vi "Elavator_Motor_Value.vi"(6 "Ele_Pos":dbl, 8 "Pos_Des":dbl, 9 "Pos_Active":bool, 11 "Ele_Manual":dbl) -> (2 "Ele_At_Pos":bool, 3 "Ele_Lift_Power":dbl)   [LabVIEW 2014]
panel:
  in  "lower limit":dbl=8.25
  in  "upper limit":dbl=53.5
  out "Pos_Power_Map":cluster{"Speed X":dbl[], "Speed Y":dbl[]}(graph)
  in  "Y_Array":dbl[](array[numeric])=[1.0, 0.15, 0.15, 0.0, -0.15, -0.15, -1.0] format="%.2f"
  in  "X_Array":dbl[](array[numeric])=[-1.75, -0.1, -0.01, 0.0, 0.01, 0.1, 1.75, 0.0, 0.0, 0.0, 100.0] format="%.2f"
  out "y_out":dbl
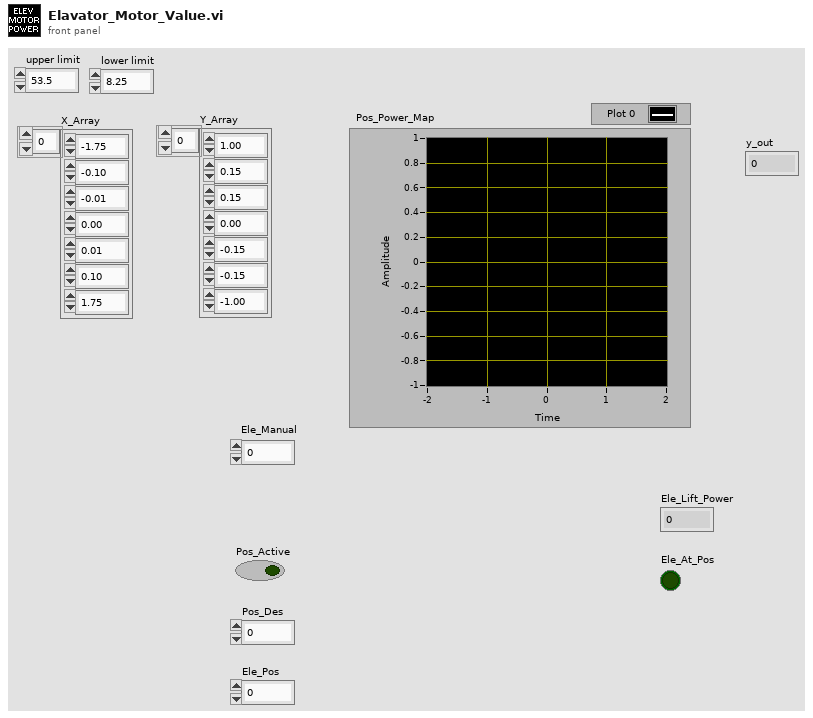
[diagram p1: front panel]
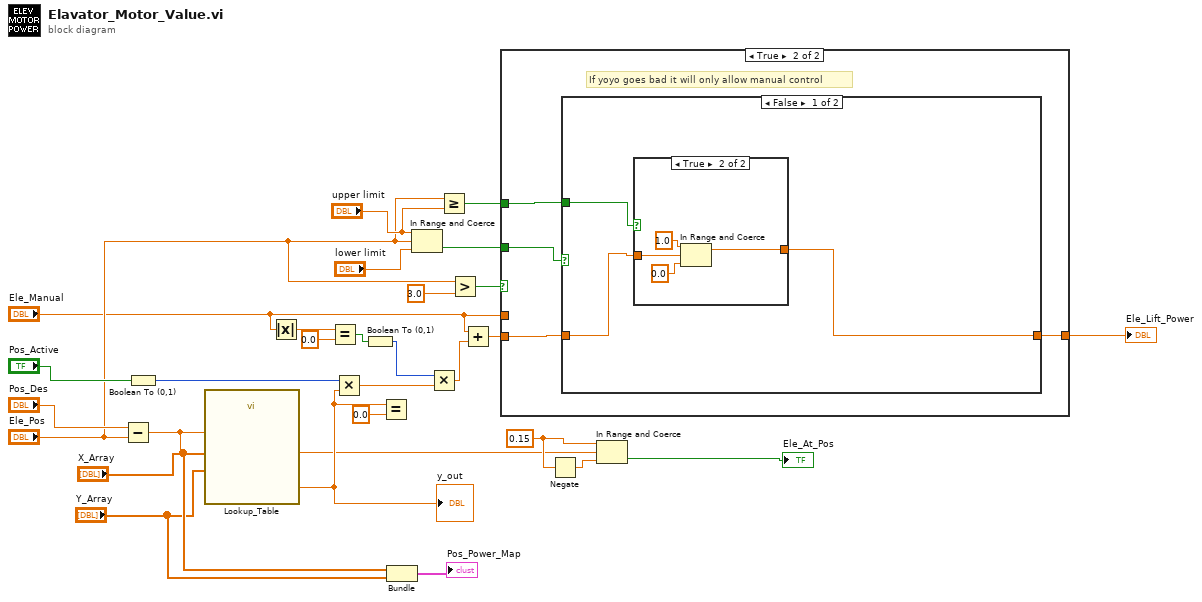
[diagram p0: block diagram]
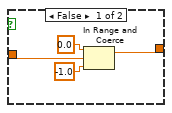
[diagram p3: hidden frame]
diagram:
  w13 = 0.15 ("upper limit")
  n1 = Subtract(x="Pos_Des", y="Ele_Pos") -> (x-y=w12:dbl)
  n2 = Boolean To (0,1)(Boolean="Pos_Active") -> (0, 1=w25:i16)
  n3 = call "Lookup_Table.vi"("Y_Array"="Y_Array", "x_in"=w12, "X_Array"="X_Array") -> ("y_out"=w18:dbl)  [unwired: 6 in]
  "y_out" <- w18
  n4 = Absolute Value(x="Ele_Manual") -> (abs(x)=w27:dbl)
  n5 = Equal?(x=w27, y=0.0) -> (x = y?=w24:bool)
  n6 = Multiply(x=w25, y=w18) -> (x*y=w22:dbl)
  n7 = Boolean To (0,1)(Boolean=w24) -> (0, 1=w23:i16)
  n8 = Equal?(x=w18, y=0.0) -> ()  [unwired: 1 out]
  n9 = Bundle("X_Array"="X_Array", "Y_Array"="Y_Array") -> (→"Pos_Power_Map":cluster{"X_Array":dbl[], "Y_Array":dbl[]})  [unwired: 1 in]
  n10 = In Range and Coerce(upper limit="upper limit", x="Ele_Pos", lower limit="lower limit") -> (In Range?=w10:bool)  [unwired: 1 out]
  n11 = Multiply(x=w23, y=w22) -> (x*y=w21:dbl)
  n12 = Greater Or Equal?(x="Ele_Pos", y="upper limit") -> (x >= y?=w6:bool)
  n13 = Greater?(x="Ele_Pos", y=3.0) -> (0:w4:bool)
  n14 = Add(x="Ele_Manual", y=w21) -> (x+y=w9:dbl)
  n15 = case shown="True" w4 {
    tunnel: w10 -> [_ w33]
    tunnel: w9 -> [_ w32]
    tunnel: [w29 w31] -> w8
    tunnel: w6 -> [_ w30]
    tunnel: "Ele_Manual" -> [w29 _]
    frame False {
      # "Failure mode"
    }
    frame True {
      # "If yoyo goes bad it will only allow manual control"
      n16 = case shown="False" w33 {
        tunnel: w32 -> [w35 w45]
        tunnel: [w34 w45] -> w31
        tunnel: w30 -> [w36 _]
        frame False {
          n17 = case shown="True" w36 {
            tunnel: w35 -> [w38 w44]
            tunnel: [w37 w41] -> w34
            frame False {
              n18 = In Range and Coerce(upper limit=0.0, x=w38, lower limit=-1.0) -> (coerced(x)=w37:dbl)  [unwired: 1 out]
            }
            frame True {
              n19 = In Range and Coerce(upper limit=1.0, x=w44, lower limit=0.0) -> (coerced(x)=w41:dbl)  [unwired: 1 out]
            }
          }
        }
        frame True {
        }
      }
    }
  }
  "Ele_Lift_Power" <- w8
  n20 = Negate(x=w13) -> (-x=w14:dbl)
  n21 = In Range and Coerce(upper limit=w13, x=w12, lower limit=w14) -> (In Range?=→"Ele_At_Pos":bool)  [unwired: 1 out]
